vi "ABR-Get Metrics.vi"(8 "error in (no error)":errorcluster, 10 "#AVERAGES":i32=1, 11 "Data in":dbl[](array[numeric])) -> (0 "error out":errorcluster, 2 "spread value":dbl, 3 "Data out":dbl[](array[numeric]))   [LabVIEW 2020]
uses:
  <vilib>/Analysis/baseanly.llb/Mean (DBL).vi
  <vilib>/gmath/NI_Gmath.lvlib
  <vilib>/Analysis/NI_AALBase.lvlib
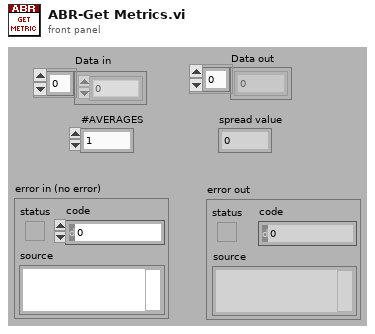
[diagram p1: front panel]
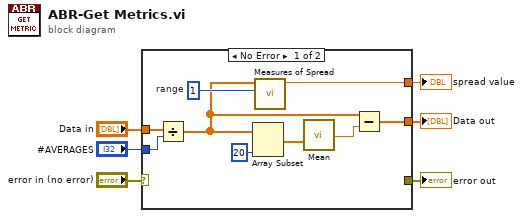
[diagram p0: block diagram]
diagram:
  n1 = case shown="No Error" "error in (no error)" {
    selector: "error in (no error)" -> [_ w16]
    tunnel: "Data in" -> [w11 _]
    tunnel: "#AVERAGES" -> [w10 _]
    tunnel: [w9 _] -> w4
    tunnel: [w7 _] -> w3
    tunnel: [_ w16] -> w1
    frame No Error {
      w12 = 1  # range
      n2 = Divide(x=w11, y=w10) -> (x/y=w8:dbl[])
      n3 = Array Subset(array=w8, length=20) -> (w13:dbl[])  [unwired: 1 in]
      n4 = call <vilib>:"Measures of Spread.vi"("type"=w12, "x array"=w8) -> ("spread value"=w7:dbl)  [unwired: 8 in, 1 out]
      n5 = call-poly <vilib>:"Mean.vi"("X"=w13) -> ("mean"=w14:dbl)  [unwired: 1 out]
      n6 = Subtract(x=w8, y=w14) -> (x-y=w9:dbl[])
    }
    frame Error {
    }
  }
  "Data out" <- w4
  "spread value" <- w3
  "error out" <- w1
